vi "Get Temperature Decline Amount.vi"(8 "Error In":errorcluster, 10 "TC Tree (AVG)":dbl, 11 "Starting Temp Decline Input":dbl) -> (0 "Error Out":errorcluster, 1 "Current Temp Decline Amout":dbl, 2 "Maximum TC Tree Temp":dbl, 3 "Starting Temp Decline Output":dbl)   [LabVIEW 2023]
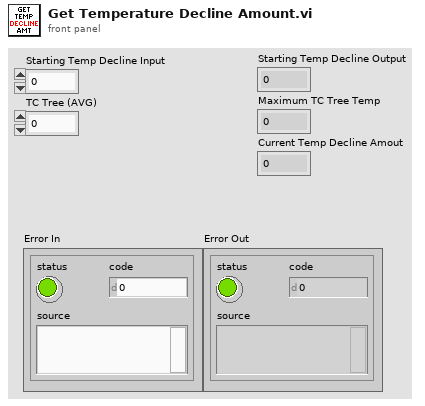
[diagram p1: front panel]
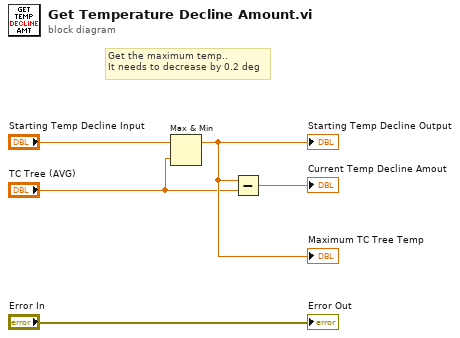
[diagram p0: block diagram]
diagram:
  # "Get the maximum temp..\nIt needs to decrease by 0.2 deg"
  n1 = Max & Min(x="Starting Temp Decline Input", y="TC Tree (AVG)") -> (max(x,y)=w5:dbl)  [unwired: 1 out]
  "Maximum TC Tree Temp" <- w5
  "Starting Temp Decline Output" <- w5
  n2 = Subtract(x=w5, y="TC Tree (AVG)") -> (x-y=→"Current Temp Decline Amout":dbl)
  "Error Out" <- "Error In"
